vi "Inovance_Set_Gain_SubVI.vi"(8 "error in (no error)":errorcluster, 9 "Gain":dbl, 11 "Refnum in":T1) -> (0 "error out":errorcluster, 1 "Gain Out":dbl)   [LabVIEW 2023, in "Inovance_Camera.lvlib"]
uses:
  Inovance_Camera.lvlib
  <resource>/objmgr/imaqdx.rc
  <vilib>/userDefined/High Color/IMAQdx.ctl
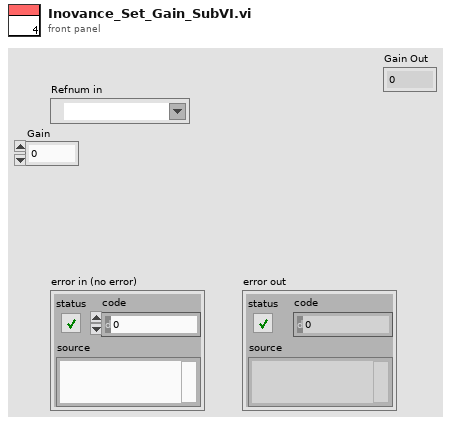
[diagram p1: front panel]
types:
  T1 = typedef "IMAQdx.ctl" = refnum<k21>
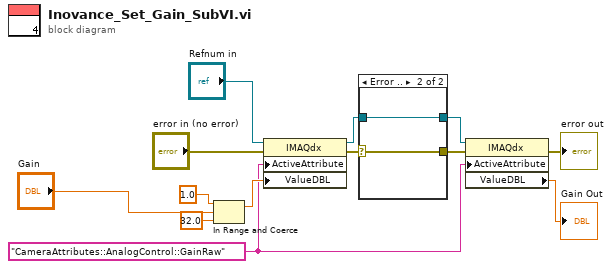
[diagram p0: block diagram]
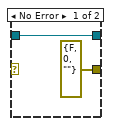
[diagram p2: hidden frame]
diagram:
  w5 = "CameraAttributes::AnalogControl::GainRaw" ("ActiveAttribute")
  n1 = In Range and Coerce(upper limit=1.0 ("y"), x="Gain", lower limit=32.0 ("y")) -> (coerced(x)=w13:dbl)  [unwired: 1 out]
  n2 = property class="IMAQdx"(reference="Refnum in", error in="error in (no error)", "ActiveAttribute"=w5, "ValueDBL"=w13) -> (reference out=w10:T1, error out=w7:errorcluster)
  n3 = case shown="Error .." w7 {
    selector: w7 -> [_ w17]
    tunnel: [errorcluster {"status"=FALSE, "code"=0, "source"=""} ("error constant") w17] -> w2
    tunnel: w10 -> [w14 w16]
    tunnel: [w14 w16] -> w6
    frame No Error {
    }
    frame Error {
    }
  }
  n4 = property class="IMAQdx"(reference=w6, error in=w2, "ActiveAttribute"=w5) -> (error out=→"error out":errorcluster, "ValueDBL"=→"Gain Out":dbl)  [unwired: 1 out]
